vi "Check_Beam_Powers.vi"(3 "Mode":T6, 5 "Traverse line In":T3 {"Row Duration (mins)" format="%#.1f"; "Row No" min=0; "Trace Gas Concentration (%)" min=0.0 format="%#.2f"; "Emission Rate (l/min)" format="%#.2f"; "Tunnel Speed" format="%#.2f"; "Start X" format="%#.2f"; "Start Y" format="%#.2f"; "Start Z" format="%#.2f"; "End X" format="%#.2f"; "End Y" format="%#.2f"; "End Z" format="%#.2f"; "Averaging time (min)" min=0.0 format="%#.2f"}) -> (0 "Error Message":string, 1 "Status":T2, 2 "Traverse line Out":T3 {"Row Duration (mins)" format="%#.1f"; "Row No" min=0; "Trace Gas Concentration (%)" min=0.0 format="%#.2f"; "Emission Rate (l/min)" format="%#.2f"; "Tunnel Speed" format="%#.2f"; "Start X" format="%#.2f"; "Start Y" format="%#.2f"; "Start Z" format="%#.2f"; "End X" format="%#.2f"; "End Y" format="%#.2f"; "End Z" format="%#.2f"; "Averaging time (min)" min=0.0 format="%#.2f"})   [LabVIEW 2012]
uses:
  Gen Trav/Traverse_cluster.ctl
  Gen Trav/Spacing.ctl
  Controls/Multi_run_mode.ctl
  Controls/User_Specific_mode.ctl
  Gen Trav/Multi_Run_Status.ctl
  Controls/Beam_Type.ctl
  Gen Trav/Route mapping/Axis.ctl
  Controls/Setup.ctl
  Controls/Save_Data.ctl
  Globals/Meas_global.vi
  Globals/Extra_Commands_Global.vi
  Globals/LDA_meas_global_1.vi
  Globals/LDA_meas_global_2.vi
panel:
  out "Light Power":dbl=8.10606551e-08 format="%^#_9e"
  in  "stop":bool
  out "Powers":dbl[](array[numeric]) format="%.4f"
  out "Beam Data":dbl[][](array[numeric]) format="%.4f"
  out "Beam Type":T1 items=["Green Unshifted", "Green Shifted", "Blue Unshifted", "Blue Shifted"]
  # "X                      Y                   Z          Datum Power"
  # "Green Unshifted\nGreen Shifted\nBlue Unshifted\nBlue Shifted"
  # "X           Y            Z"
  # "Start"
  # "End"
  # "X           Y            Z"
  # "Start"
  # "End"
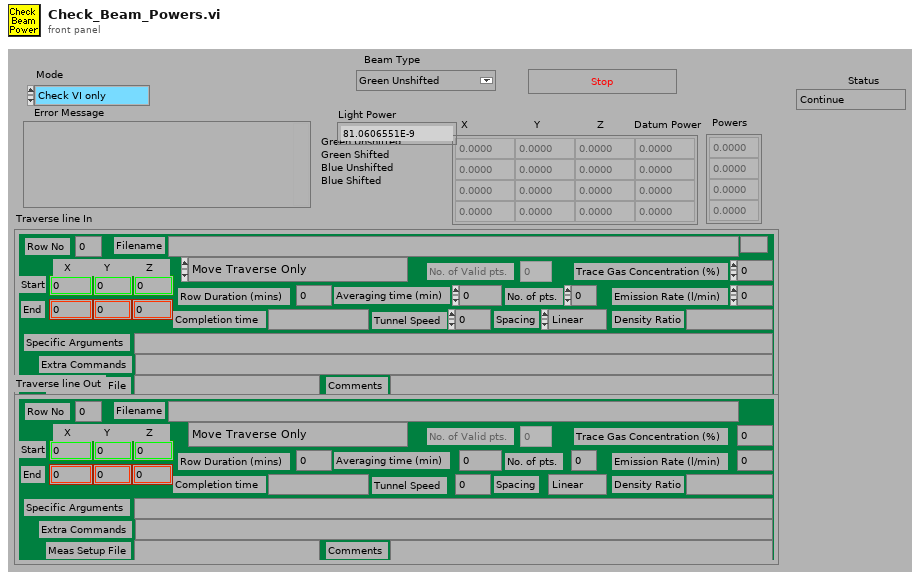
[diagram p1: front panel]
types:
  T1 = typedef "Beam_Type.ctl" = u16
  T2 = typedef "Multi_Run_Status.ctl" = enum16{"Continue", "Jump to Next Point", "Jump to Next Row", "Jump To Fall Back", "Terminate Run"}
  T3 = typedef "Traverse_cluster.ctl" = cluster{"Start X":dbl, "Start Y":dbl, "Start Z":dbl, "End X":dbl, "End Y":dbl, "End Z":dbl, "No. of pts.":i32, "Spacing":T4, "Filename":path, "Tunnel Speed":dbl, "Averaging time (min)":dbl, "Extra Commands":string, "Specific Arguments":string, "Emission Rate (l/min)":dbl, "Trace Gas Concentration (%)":dbl, "Density Ratio":string, "Comments":string, "Row No":i32, "Row Type Selector":T5, "Completion time":string, "Row Duration (mins)":dbl, "No. of Valid pts.":i32, "Meas Setup File":string}
  T4 = typedef "Spacing.ctl" = enum16{"Linear", "Log", "Gauss", "Specified", "N/A"}
  T5 = typedef "Multi_run_mode.ctl" = enum16{"Move Traverse Only", "Set Tunnel Speed Only", "Set Source Only", "Set Measurement Conditions", "Single Measurement", "Vertical Profile", "Lateral Profile", "Longitudinal Profile", "Explore Volume", "Multi-Axis Profile", "Auto Calibrate", "Meas Fast FID Bkgnd", "Check Beam Power", "Scanning Valve Measurement", "Run VI Named:", "Set ADAM Ch", "Wait (minutes)", "Send Message", "Synchronize With:", "Fall Back to this Row", "Turn Off Row Repeating", "Blank Row", "Traverse 3D Volume"}
  T6 = typedef "User_Specific_mode.ctl" = enum16{"Check VI only", "Run VI"}
  T7 = enum32{"Bad", "Idle", "Run top level", "Running"}
  T8 = typedef "LDA_Setup.ctl" = cluster{"dimensions":enum16{"1D", "2D"}, "Analogue Freq Multiplier":dbl}
  T9 = enum16{"Load From Excel File", "Save to Excel File"}
  T10 = typedef "Axis.ctl" = enum16{"X Axis", "X Axis -ve", "Y Axis", "Y Axis -ve", "Z Axis", "Z Axis -ve"}
  T11 = typedef "Save_Data.ctl" = enum16{"Save No Data", "Save Data"}
  T12 = typedef "Setup.ctl" = enum16{"Run Program", "Show Setup", "Save Current Setup", "Setup Front Panel"}
  T13 = typedef "Status_Cluster.ctl" = cluster{"Status":T2, "Error Type":string, "Error Description":string}
  T14 = typedef "BSA_Type.ctl" = enum16{"57N11", "BSA F60"}
  T15 = typedef "BSA_info_Cluster.ctl" = cluster{"GPIB Address":string, "No of Check Bytes":i32, "Extra Info":string, "COLOUR":u32, "Wavelength (nm)":dbl}
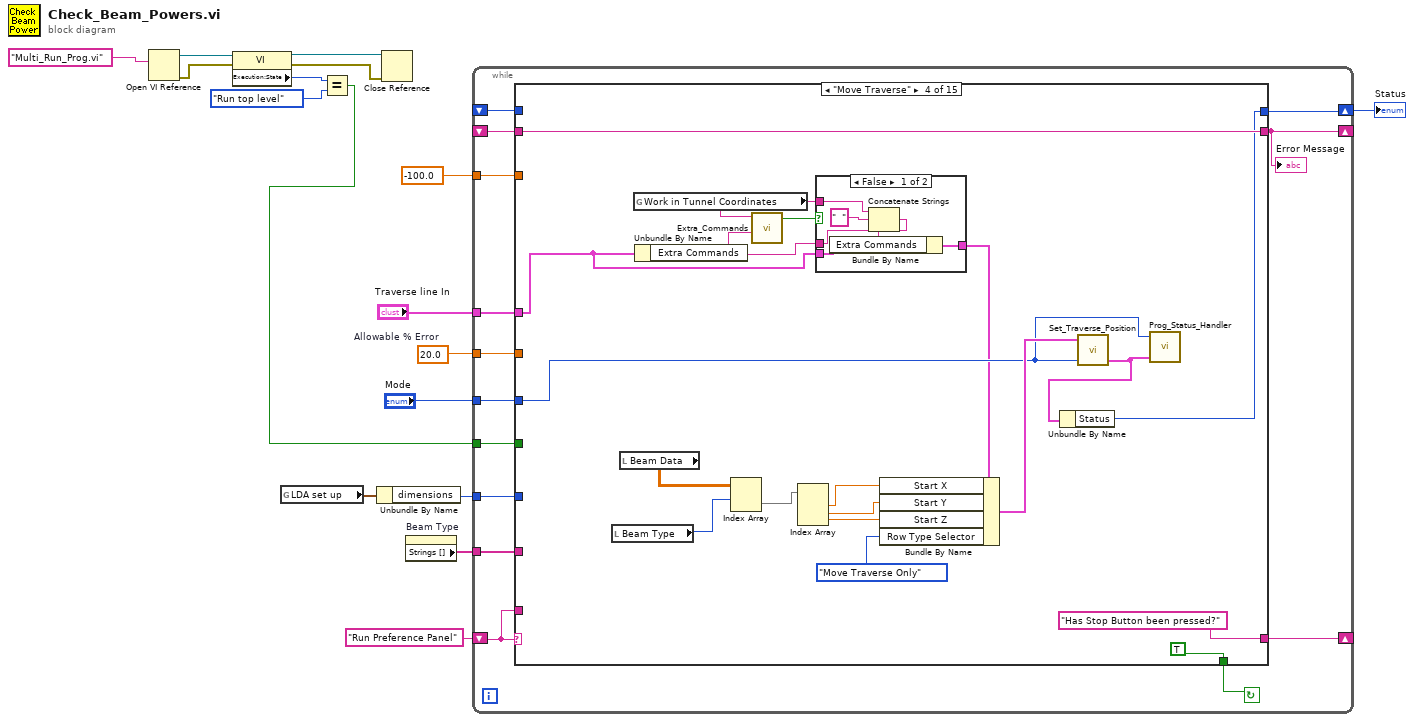
[diagram p0: block diagram]
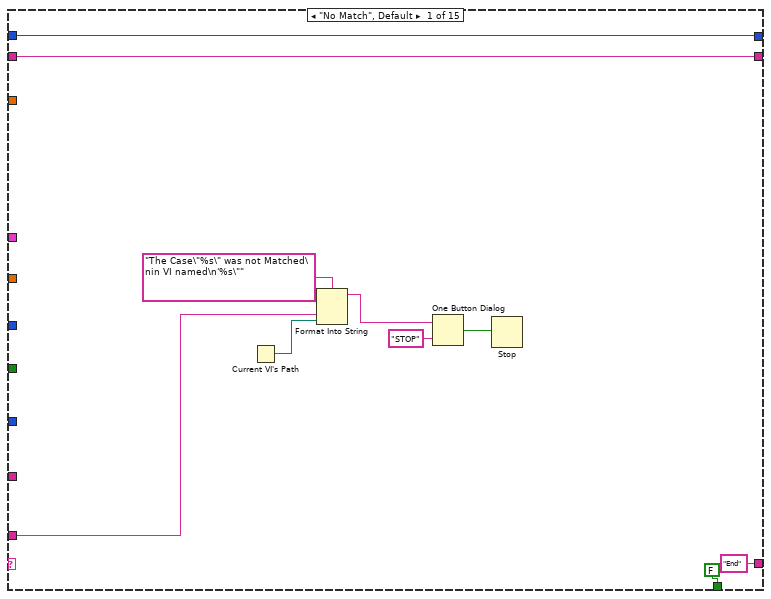
[diagram p2: hidden frame]
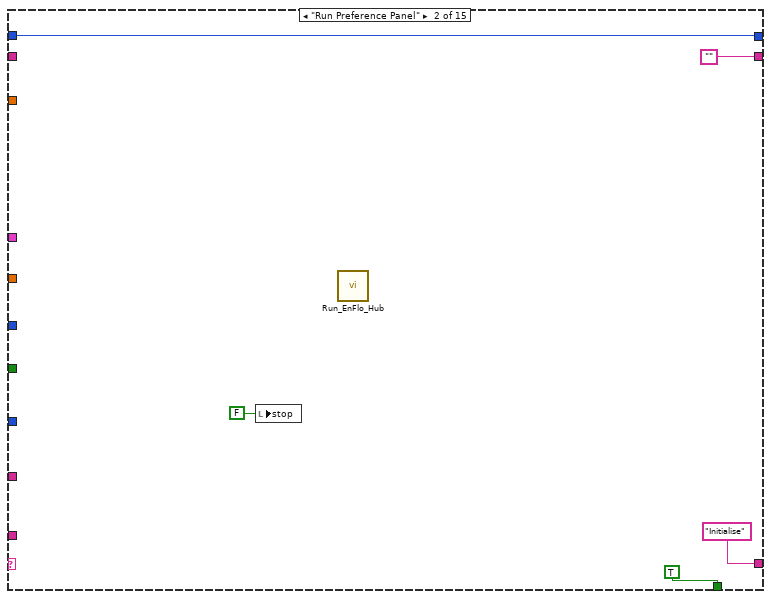
[diagram p3: hidden frame]
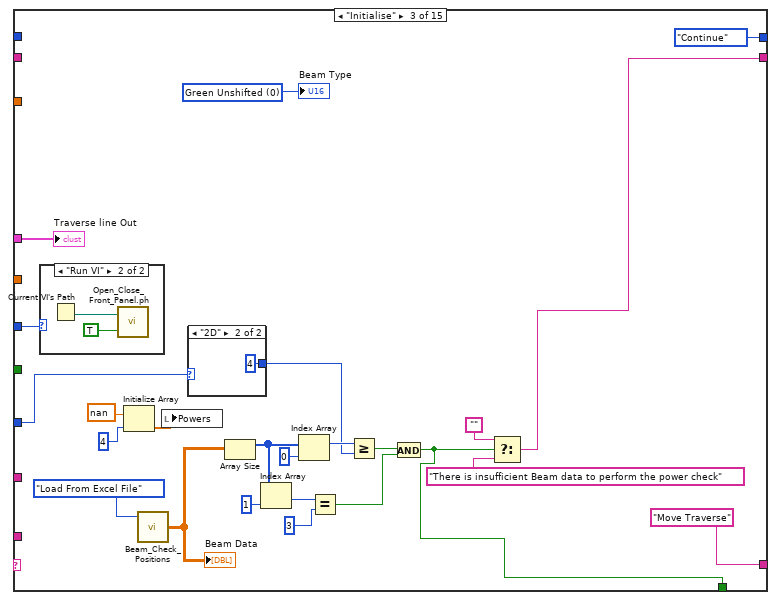
[diagram p4: hidden frame]
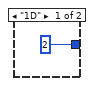
[diagram p5: hidden frame]
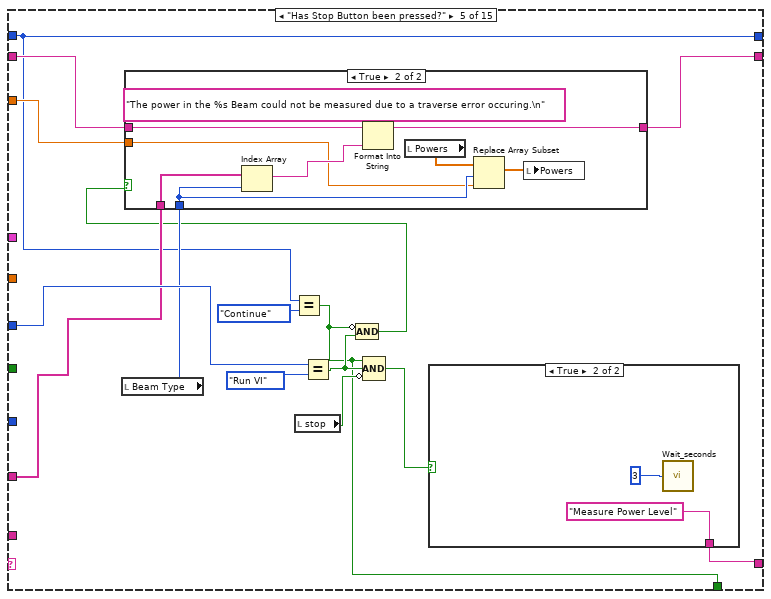
[diagram p8: hidden frame]
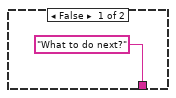
[diagram p10: hidden frame]
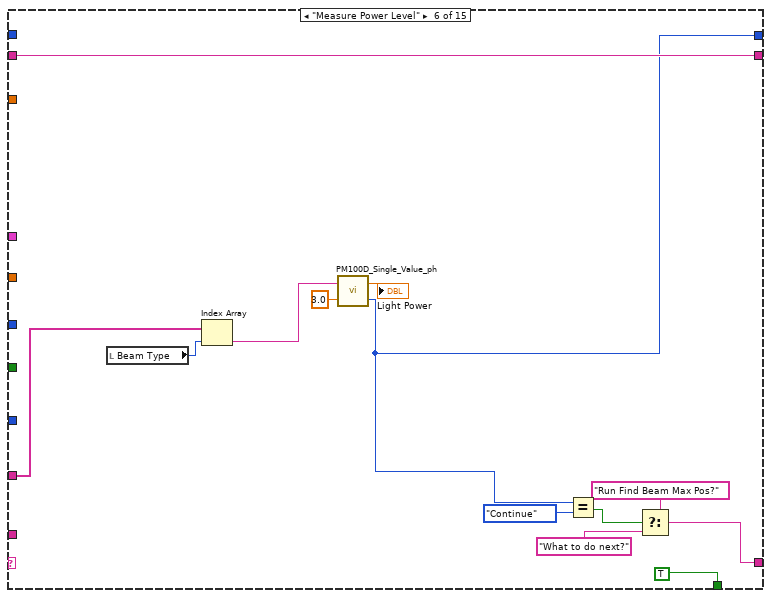
[diagram p11: hidden frame]
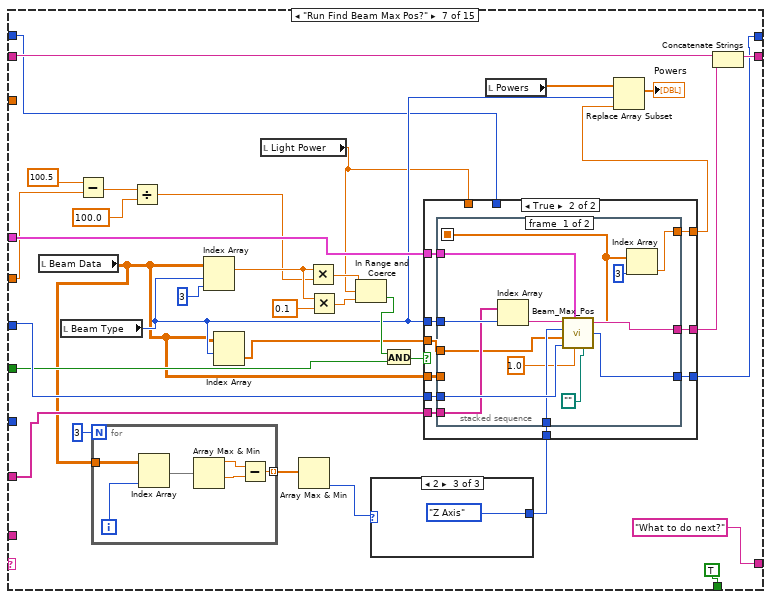
[diagram p12: hidden frame]
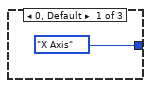
[diagram p13: hidden frame]
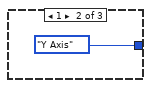
[diagram p14: hidden frame]
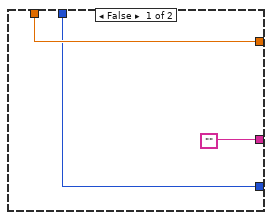
[diagram p15: hidden frame]
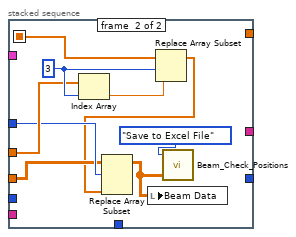
[diagram p16: hidden frame]
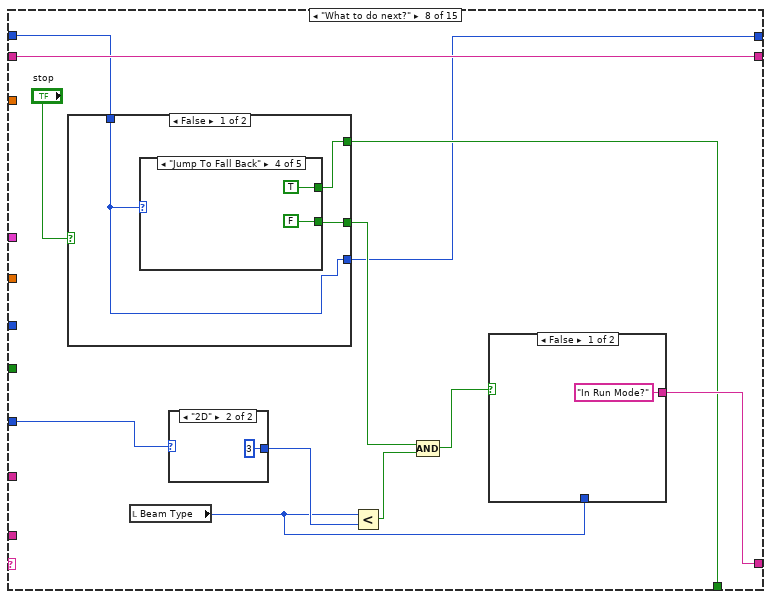
[diagram p17: hidden frame]
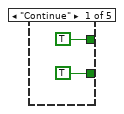
[diagram p18: hidden frame]
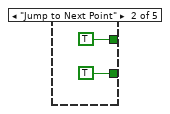
[diagram p19: hidden frame]
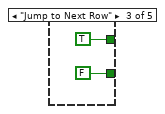
[diagram p20: hidden frame]
diagram:
  w14 = 20.0  # Allowable % Error
  n1 = Open VI Reference(vi path="Multi_Run_Prog.vi") -> (vi reference=w8:refnum<vi>, error out=w9:errorcluster)  [unwired: 1 in, 4 out]
  n2 = property class="VI"(reference=w8, error in=w9) -> (reference out=w10:refnum<vi>, error out=w11:errorcluster, "Execution:State"=w7:T7)
  n3 = global read "Meas_global.vi" "LDA set up"() -> (w2:T8)
  n4 = Equal?(x=w7, y=T7."Run top level" ("Exec.State")) -> (x = y?=w5:bool)
  n5 = Unbundle By Name(w2) -> ("dimensions"=w1:enum16{"1D", "2D"})
  n6 = Close Reference(reference=w10, error in (no error)=w11) -> ()  [unwired: 1 out]
  n7 = property on="Beam Type" class="Ring (strict)"() -> ("Strings []"=w15:string[])  [unwired: 2 in, 2 out]
  n8 = while {
    tunnel: -100.0 ("Element Data") -> [w21]
    tunnel: w14 -> [w23]
    shift-left: _ -> [w25]
    shift-right: [w24] -> _
    tunnel: w1 -> [w26]
    tunnel: w15 -> [w29]
    tunnel: "Traverse line In" -> [w30]
    tunnel: "Mode" -> [w31]
    shift-left: "Run Preference Panel" -> [w22]
    shift-right: [w27] -> _
    tunnel: w5 -> [w20]
    shift-right: [w19] -> w3
    shift-left: _ -> [w18]
    stop <- w28 continue-if-true
    n9 = case shown="\"Move Traverse\"" w22 {
      tunnel: w30 -> [_ _ w68 w76 _ _ w174 _ _ _ _ _ _ w364 _]
      tunnel: w31 -> [_ _ w65 w89 w113 _ w173 _ w262 _ _ _ _ w368 w373]
      tunnel: w29 -> [_ _ _ _ w111 w131 w148 _ _ w279 _ _ _ _ _]
      tunnel: [FALSE ("Update Datum Powers?") TRUE ("Update Datum Powers?") w47 TRUE w102 TRUE TRUE w223 TRUE ("Update Datum Powers?") TRUE TRUE TRUE ("Update Datum Powers?") w334 w365 FALSE ("Update Datum Powers?")] -> w28
      tunnel: ["End" "Initialise" "Move Traverse" "Has Stop Button been pressed?" w112 w136 "What to do next?" w225 w257 "Log Beam Power Readings" w311 "Take datum velocity measurement?" "Move traverse to datum location" "Take a datum velocity measurement" "End"] -> w27
      tunnel: w26 -> [_ _ w64 _ _ _ _ w231 _ _ _ _ w336 _ _]
      tunnel: w25 -> [w33 _ _ w87 w109 w138 w160 w227 w261 w277 w306 w325 w338 w370 w376]
      tunnel: [w33 "" w48 w87 w110 w138 w159 w227 w261 w276 w306 "" w338 w370 w376] -> w24
      tunnel: w23 -> [_ _ _ _ _ _ w156 _ _ _ _ _ _ _ _]
      tunnel: w22 -> [w36 _ _ _ _ _ _ _ _ _ _ _ _ _ _]
      tunnel: w21 -> [_ _ _ _ w108 _ _ _ _ w274 _ _ _ _ _]
      tunnel: w20 -> [_ _ _ _ _ _ w149 _ _ _ _ _ w333 _ _]
      tunnel: [w32 w42 Multi_Run_Status."Continue" ("Status") w84 w101 w133 w143 w221 w255 w273 w309 w321 w331 w363 w372] -> w19
      tunnel: w18 -> [w32 w42 _ _ w101 _ w142 w222 w255 w273 w309 w321 w331 _ w371]
      frame "No Match", Default {
        n10 = Current VI's Path() -> (path=w37:path)
        n11 = Format Into String(format string="The Case\"%s\" was not Matched\nin VI named\n'%s\"" ("Format String"), w36, w37) -> (resulting string=w40:string)  [unwired: 2 in, 1 out]
        n12 = One Button Dialog(message=w40, button name ("OK")="STOP") -> (true=w38:bool)
        n13 = Stop(stop? (T)=w38) -> ()
      }
      frame "Run Preference Panel" {
        n14 = local write "stop"(FALSE ("stop")) -> ()
        n15 = call "Run_EnFlo_Hub.vi"() -> ()  [unwired: 8 out]
      }
      frame "Initialise" {
        w69 = T1 0 items=["Green Unshifted", "Green Shifted", "Blue Unshifted", "Blue Shifted"] ("Beam Type")
        n16 = case shown="\"Run VI\"" w65 {
          frame "Check VI only" {
          }
          frame "Run VI" {
            n17 = Current VI's Path() -> (path=w73:path)
            n18 = call "Open_Close_Front_Panel.ph.vi"("Front Panel Window:Open"=TRUE, "VI path"=w73) -> ()  [unwired: 2 out]
          }
        }
        n19 = Initialize Array(nan ("Numeric"), 4 ("Dimension Size")) -> (w51:dbl[])
        n20 = call "Beam_Check_Positions.vi"("Mode"=T9."Load From Excel File") -> ("Values Out"=w67:dbl[][])  [unwired: 1 in, 1 out]
        "Beam Data" <- w67
        n21 = local write "Powers"(w51) -> ()
        n22 = case shown="\"2D\"" w64 {
          tunnel: [2 4] -> w62
          frame "1D" {
          }
          frame "2D" {
          }
        }
        n23 = Array Size(array=w67) -> (size(s)=w58:i32[])
        n24 = Index Array(array=w58, index=1 ("Index")) -> (element=w57:i32)
        n25 = Index Array(array=w58, index=0 ("Index")) -> (element=w63:i32)
        n26 = Equal?(x=w57, y=3) -> (x = y?=w54:bool)
        n27 = Greater Or Equal?(x=w63, y=w62) -> (x >= y?=w55:bool)
        n28 = And(x=w55, y=w54) -> (x .and. y?=w47:bool)
        n29 = Select(t="", s=w47, f="There is insufficient Beam data to perform the power check") -> (s? t:f=w48:string)
        "Beam Type" <- w69
        "Traverse line Out" <- w68
      }
      frame "Move Traverse" {
        n30 = local read "Beam Type"() -> (w85:T1)
        n31 = local read "Beam Data"() -> (w86:dbl[][])
        n32 = global read "Extra_Commands_Global.vi" "Work in Tunnel Coordinates"() -> (w78:string)
        n33 = Unbundle By Name(w76) -> ("Extra Commands"=w77:string)
        n34 = Index Array(array=w86, index (row)=w85) -> (element=w83:dbl[])  [unwired: 1 in]
        n35 = call "Extra_Commands.vi"("String to Search"=w77, "Command"=w78) -> ("Command Found"=w79:bool)  [unwired: 1 in, 4 out]
        n36 = Index Array(array=w83) -> (element #1=w82:dbl, element #2=w81:dbl, element #3=w80:dbl)  [unwired: 3 in]
        n37 = case shown="False" w79 {
          tunnel: [w99 w100] -> w75
          tunnel: w78 -> [w98 _]
          tunnel: w77 -> [w97 _]
          tunnel: w76 -> [w95 w100]
          frame False {
            n38 = Concatenate Strings(w98, "  " ("string"), w97) -> (w96:string)
            n39 = Bundle By Name(cluster=w95, "Extra Commands"=w96) -> (w99:T3)
          }
          frame True {
          }
        }
        n40 = Bundle By Name(cluster=w75, "Start X"=w82, "Start Y"=w81, "Start Z"=w80, "Row Type Selector"=Multi_run_mode."Move Traverse Only") -> (w92:T3)
        n41 = call "Set_Traverse_Position.vi"("Simulate/Run"=w89, "Traverse line"=w92) -> ("Status Cluster"=w90:T13)  [unwired: 1 in, 2 out]
        n42 = Unbundle By Name(w90) -> ("Status"=w84:T2)
        n43 = call "Prog_Status_Handler.vi"("Status Cluster"=w90, "Simulate/Run"=w89) -> ()  [unwired: 2 out]
      }
      frame "Has Stop Button been pressed?" {
        n44 = local read "Beam Type"() -> (w107:T1)
        n45 = Equal?(x=w101, y=Multi_Run_Status."Continue" ("Status")) -> (x = y?=w102:bool)
        n46 = local read "stop"() -> (w106:bool)
        n47 = Equal?(x=w113, y=User_Specific_mode."Run VI" ("Mode")) -> (x = y?=w104:bool)
        n48 = Compound Arithmetic op=AND(invert w102, w104) -> (w103:bool)
        n49 = case shown="True" w103 {
          tunnel: w107 -> [_ w118]
          tunnel: w111 -> [_ w125]
          tunnel: w109 -> [w116 w122]
          tunnel: [w116 w121] -> w110
          tunnel: w108 -> [_ w117]
          frame False {
          }
          frame True {
            n50 = Index Array(array=w125, index=w118) -> (element=w124:string)
            n51 = Format Into String(format string="The power in the %s Beam could not be measured due to a traverse error occuring.\n" ("Format String"), initial string=w122, w124) -> (resulting string=w121:string)  [unwired: 1 in, 1 out]
            n52 = local read "Powers"() -> (w120:dbl[])
            n53 = Replace Array Subset(array=w120, new element=w117, index=w118) -> (w119:dbl[])
            n54 = local write "Powers"(w119) -> ()
          }
        }
        n55 = Compound Arithmetic op=AND(w102, w104, invert w106) -> (w105:bool)
        n56 = case shown="True" w105 {
          tunnel: ["What to do next?" "Measure Power Level"] -> w112
          frame False {
          }
          frame True {
            n57 = call "Wait_seconds.vi"("Seconds to wait"=u32 3) -> ()
          }
        }
      }
      frame "Measure Power Level" {
        n58 = local read "Beam Type"() -> (w132:T1)
        n59 = Index Array(array=w131, index=w132) -> (element=w130:string)
        n60 = call "PM100D_Single_Value_ph.vi"("Averaging Period (s)"=3.0, "Beam Name"=w130) -> ("Status"=w133:T2, "Light Power mW"=→"Light Power":dbl)
        n61 = Equal?(x=w133, y=Multi_Run_Status."Continue" ("Status")) -> (x = y?=w139:bool)
        n62 = Select(t="Run Find Beam Max Pos?", s=w139, f="What to do next?") -> (s? t:f=w136:string)
      }
      frame "Run Find Beam Max Pos?" {
        n63 = local read "Beam Data"() -> (w145:dbl[][])
        n64 = local read "Beam Type"() -> (w147:T1)
        n65 = Subtract(x=100.5, y=w156) -> (x-y=w155:dbl)
        n66 = for {
          N: 3 -> [_]
          tunnel: w145 -> [w183]
          tunnel: [w179] -> w171 mode=indexing
          i -> [w184]
          n67 = Index Array(array=w183, index (col)=w184) -> (element=w182:dbl[])  [unwired: 1 in]
          n68 = Array Max & Min(array=w182) -> (max value=w181:dbl, min value=w180:dbl)  [unwired: 2 out]
          n69 = Subtract(x=w181, y=w180) -> (x-y=w179:dbl)
        }
        n70 = Divide(x=w155, y=100.0) -> (x/y=w153:dbl)
        n71 = Index Array(array=w145, index (row)=w147, index (col)=3 ("Index")) -> (element=w167:dbl)
        n72 = Index Array(array=w145, index (row)=w147) -> (element=w146:dbl[])  [unwired: 1 in]
        n73 = local read "Light Power"() -> (w144:dbl)
        n74 = Array Max & Min(array=w171) -> (min index (indices)=w170:i32)  [unwired: 3 out]
        n75 = Multiply(x=w167, y=w153) -> (x*y=w165:dbl)
        n76 = Multiply(x=w167, y=0.1) -> (x*y=w164:dbl)
        n77 = In Range and Coerce(upper limit=w165, x=w144, lower limit=w164) -> (In Range?=w151:bool)  [unwired: 1 out]
        n78 = case shown="2" w170 {
          tunnel: [Axis."X Axis" ("Fixed Axis") Axis."Y Axis" ("Fixed Axis") Axis."Z Axis" ("Fixed Axis")] -> w169
          frame 0, Default {
          }
          frame 1 {
          }
          frame 2 {
          }
        }
        n79 = And(x=w151, y=w149) -> (x .and. y?=w150:bool)
        n80 = case shown="True" w150 {
          tunnel: w147 -> [_ w192]
          tunnel: w174 -> [_ w197]
          tunnel: w173 -> [_ w196]
          tunnel: w169 -> [_ w195]
          tunnel: [w187 w194] -> w161
          tunnel: w144 -> [w187 _]
          tunnel: ["" w193] -> w158
          tunnel: w148 -> [_ w191]
          tunnel: w146 -> [_ w190]
          tunnel: w145 -> [_ w189]
          tunnel: [w185 w188] -> w143
          tunnel: w142 -> [w185 _]
          frame False {
          }
          frame True {
            n81 = stacked-sequence {
              seq-local: [w200 _] -> [_ w218]
              tunnel: w197 -> [w211 _]
              tunnel: w196 -> [w210 _]
              tunnel: w195 -> [w209 _]
              tunnel: [w207 _] -> w194
              tunnel: [w206 _] -> w193
              tunnel: w192 -> [w204 w216]
              tunnel: w191 -> [w203 _]
              tunnel: w190 -> [w201 w217]
              tunnel: w189 -> [_ w215]
              tunnel: [w198 _] -> w188
              frame #0 {
                n82 = Index Array(array=w203, index=w204) -> (element=w202:string)
                n83 = call "Beam_Max_Pos.vi"("Picture Log"=path "", "Search Step (mm)"=1.0, "Mode"=w210, "Starting Position"=w201, "Traverse line In"=w211, "Fixed Axis"=w209, "Beam Name"=w202) -> ("Status"=w198:T2, "Beam maxima"=w200:dbl[], "Message"=w206:string)  [unwired: 1 out]
                n84 = Index Array(array=w200, index=3 ("Index")) -> (element=w207:dbl)
              }
              frame #1 {
                w219 = 3 ("index")
                n85 = Index Array(array=w217, index=w219) -> (element=w220:dbl)
                n86 = Replace Array Subset(array=w218, new element=w220, index=w219) -> (w212:dbl[])
                n87 = Replace Array Subset(array=w215, new element=w212, index (row)=w216) -> (w214:dbl[][])  [unwired: 1 in]
                n88 = local write "Beam Data"(w214) -> ()
                n89 = call "Beam_Check_Positions.vi"("Values"=w214, "Mode"=T9."Save to Excel File") -> ()  [unwired: 2 out]
              }
            }
          }
        }
        n90 = local read "Powers"() -> (w163:dbl[])
        n91 = Replace Array Subset(array=w163, new element=w161, index=w147) -> (→"Powers":dbl[])
        n92 = Concatenate Strings(w160, w158) -> (w159:string)
      }
      frame "What to do next?" {
        n93 = case shown="False" "stop" {
          tunnel: [w235 FALSE] -> w224
          tunnel: [w234 FALSE] -> w223
          tunnel: w222 -> [w233 _]
          tunnel: [w233 Multi_Run_Status."Terminate Run" ("Status")] -> w221
          frame False {
            n94 = case shown="\"Jump To Fall Back\"" w233 {
              tunnel: [TRUE TRUE FALSE FALSE FALSE] -> w235
              tunnel: [TRUE TRUE TRUE TRUE FALSE] -> w234
              frame "Continue" {
              }
              frame "Jump to Next Point" {
              }
              frame "Jump to Next Row" {
              }
              frame "Jump To Fall Back" {
              }
              frame "Terminate Run" {
              }
            }
          }
          frame True {
          }
        }
        n95 = local read "Beam Type"() -> (w228:T1)
        n96 = case shown="\"2D\"" w231 {
          tunnel: [1 3] -> w232
          frame "1D" {
          }
          frame "2D" {
          }
        }
        n97 = Less?(x=w228, y=w232) -> (x < y?=w230:bool)
        n98 = Compound Arithmetic op=AND(w224, w230) -> (w229:bool)
        n99 = case shown="False" w229 {
          tunnel: w228 -> [_ w252]
          tunnel: ["In Run Mode?" "Move Traverse"] -> w225
          frame False {
          }
          frame True {
            n100 = Increment(x=w252) -> (x+1=w251:T1)
            n101 = local write "Beam Type"(w251) -> ()
          }
        }
      }
      frame "In Run Mode?" {
        n102 = Equal?(x=w262, y=User_Specific_mode."Run VI" ("Mode")) -> (x = y?=w259:bool)
        n103 = Select(t="Are Powers Acceptable?", s=w259, f="Move traverse to datum location") -> (s? t:f=w257:string)
      }
      frame "Are Powers Acceptable?" {
        n104 = global read "LDA_meas_global_1.vi" "Min Green Unshifted Power mW"() -> (w265:i32)
        n105 = global read "LDA_meas_global_1.vi" "Min Blue Unshifted Power mW"() -> (w267:i32)
        n106 = global read "LDA_meas_global_1.vi" "Min Green Shifted Power mW"() -> (w266:i32)
        n107 = global read "LDA_meas_global_1.vi" "Min Blue Shifted Power mW"() -> (w268:i32)
        n108 = local read "Powers"() -> (w280:dbl[])
        n109 = Build Array(w265, w266, w267, w268) -> (w269:i32[])
        n110 = To Double Precision Float(number=w269) -> (double precision float=w264:dbl[])
        n111 = for {
          tunnel: w280 -> [w287] mode=indexing
          tunnel: w264 -> [w286] mode=indexing
          shift-right: [w296] -> w271
          shift-left: "" -> [w298]
          tunnel: w279 -> [w297] mode=indexing
          tunnel: w274 -> [w291]
          n112 = Subtract(x=w287, y=w286) -> (x-y=w292:dbl)
          n113 = Divide(x=w292, y=w286) -> (x/y=w294:dbl)
          n114 = Not Equal?(x=w291, y=w287) -> (x != y?=w288:bool)
          n115 = Absolute Value(x=w294) -> (abs(x)=w293:dbl)
          n116 = Multiply(x=w293, y=100.0) -> ()  [unwired: 1 out]
          n117 = Less Than 0?(x=w292) -> (x < 0?=w289:bool)
          n118 = Compound Arithmetic op=AND(w288, w289) -> (w290:bool)
          n119 = case shown="True" w290 {
            tunnel: w298 -> [w299 w304]
            tunnel: w297 -> [_ w305]
            tunnel: [w299 w303] -> w296
            tunnel: w287 -> [_ w301]
            tunnel: w286 -> [_ w300]
            frame False {
            }
            frame True {
              n120 = Format Into String(format string="The %s laser beam power is %.1f mW. It lowest acceptable power has been set to %.1f mW. \\n" ("Format String"), initial string=w304, w305, w301, w300) -> (resulting string=w303:string)  [unwired: 1 in, 1 out]
            }
          }
        }
        n121 = Empty String/Path?(string/path=w271) -> (empty?=w272:bool)
        n122 = case shown="False" w272 {
          tunnel: w271 -> [w283 w285]
          tunnel: [w282 w285] -> w270
          frame False {
            n123 = Concatenate Strings(w283, "Please come and check the system As Soon As Possible!\nThe probe may have collided with something or the optical fibres could be getting damaged due to poor launch efficiency! £18,000 TO REPAIR!!\nThe Multi Run will continue." ("Substring")) -> (w282:string)
          }
          frame True {
          }
        }
        n124 = Concatenate Strings(w277, w270) -> (w276:string)
      }
      frame "Log Beam Power Readings" {
        n125 = local read "Beam Data"() -> (w314:dbl[][])
        n126 = local read "Powers"() -> (w313:dbl[])
        n127 = for {
          tunnel: w314 -> [w320] mode=indexing
          tunnel: w313 -> [w317] mode=indexing
          tunnel: [w316] -> w312 mode=indexing
          n128 = Array Subset(array=w320, length=3 ("Array Length")) -> (w318:dbl[])  [unwired: 1 in]
          n129 = Build Array (concatenate)(w318, w317) -> (w316:dbl[])
        }
        n130 = Empty String/Path?(string/path=w306) -> (empty?=w307:bool)
        n131 = call "Log_beam_power.vi"("Message"=w306, "Beam Data"=w312) -> ()  [unwired: 4 out]
        n132 = Select(t="Take datum velocity measurement?", s=w307, f="Send Error Email") -> (s? t:f=w311:string)
      }
      frame "Send Error Email" {
        w329 = FALSE  # Dialog Box (T)
        n133 = Bundle By Name(cluster=errorcluster {"status"=FALSE, "code"=0, "source"=""} ("error in (no error)"), "source"=w325, "status"=TRUE ("Bundle Element")) -> (w327:errorcluster)
        n134 = call "EnFlo_Error_Handler.vi"("error in (no error)"=w327, "Error Type"="Beam Power", "Dialog Box (T)"=w329) -> ()  [unwired: 3 out]
      }
      frame "Take datum velocity measurement?" {
        n135 = global read "LDA_meas_global_1.vi" "BSA Type"() -> (w332:T14)
        n136 = case shown="\"57N11\"" w332 {
          tunnel: w336 -> [w341 _]
          tunnel: [w340 TRUE] -> w335
          tunnel: w333 -> [w339 _]
          frame "57N11" {
            n137 = stacked-sequence {
              tunnel: w341 -> [_ w354]
              tunnel: [_ w350] -> w340
              tunnel: w339 -> [w342 _]
              frame #0 {
                n138 = case shown="True" w342 {
                  frame False {
                  }
                  frame True {
                    n139 = stacked-sequence {
                      frame #0 {
                        n140 = global read "LDA_meas_global_2.vi" "BSA2 info"() -> (w343:T15)
                        n141 = global read "LDA_meas_global_1.vi" "BSA1 info"() -> (w348:T15)
                        n142 = Unbundle By Name(w343) -> ("GPIB Address"=w344:string)
                        n143 = Unbundle By Name(w348) -> ("GPIB Address"=w347:string)
                        n144 = call "Set_BSA_voltage_On_Off.vi"("GPIB address"=w344, "High Voltage"=TRUE) -> ()  [unwired: 1 in, 5 out]
                        n145 = call "Set_BSA_voltage_On_Off.vi"("GPIB address"=w347, "High Voltage"=TRUE) -> ()  [unwired: 1 in, 5 out]
                      }
                      frame #1 {
                        n146 = call "Wait_seconds.vi"("Seconds to wait"=u32 5) -> ()
                      }
                    }
                  }
                }
              }
              frame #1 {
                w351 = 7.0 ("y")
                n147 = call "LDA_data_rate.vi"() -> ("Data rate (Hz) BSA1"=w355:dbl, "Data rate (Hz) BSA2"=w352:dbl)  [unwired: 1 out]
                n148 = Greater?(x=w355, y=w351) -> (0:w353:bool)
                n149 = case shown="\"1D\"" w354 {
                  tunnel: w353 -> [w356 w360]
                  tunnel: w352 -> [_ w359]
                  tunnel: w351 -> [_ w358]
                  tunnel: [w356 w357] -> w350
                  frame "1D" {
                  }
                  frame "2D" {
                    n150 = Greater?(x=w359, y=w358) -> (0:w361:bool)
                    n151 = And(x=w360, y=w361) -> (x .and. y?=w357:bool)
                  }
                }
              }
            }
          }
          frame "BSA F60" {
          }
        }
        n152 = And(x=w335, y=w333) -> (x .and. y?=w334:bool)
      }
      frame "Move traverse to datum location" {
        n153 = call "Set_Traverse_Position.vi"("Simulate/Run"=w368, "Traverse line"=w364) -> ("Status Cluster"=w367:T13)  [unwired: 1 in, 2 out]
        n154 = Unbundle By Name(w367) -> ("Status"=w363:T2)
        n155 = Equal?(x=Multi_Run_Status."Continue" ("Status"), y=w363) -> (x = y?=w365:bool)
      }
      frame "Take a datum velocity measurement" {
        n156 = case shown="\"Run VI\"" w373 {
          tunnel: [w377 w378] -> w372
          tunnel: w371 -> [w377 _]
          frame "Check VI only" {
          }
          frame "Run VI" {
            n157 = flat-sequence {
              tunnel: [w383] -> w380
              tunnel: [w382] -> w379
              tunnel: [w381] -> w378
              tunnel: w380 -> [w391]
              tunnel: w379 -> [w390]
              frame #0 {
                w385 = 1.0  # Averaging time (min)
                w388 = FALSE  # Open Front Panel
                w389 = FALSE  # Remote control
                n158 = call "Create_Error_log_folders.vi"("Log Filename"="LDA_Datum_Vel.xls" ("Input Element")) -> ("Server copy Location"=w382:path, "Local Log File"=w383:path)  [unwired: 2 in, 1 out]
                n159 = call "Code_to_run.vi"("Open Front Panel"=w388, "setup"=Setup."Run Program", "Remote control"=w389, "File"=Save_Data."Save Data", "Results Filename"=w383, "Averaging time (min)"=w385) -> ("Status"=w381:T2)  [unwired: 5 in, 4 out]
              }
              frame #1 {
                n160 = call "Updated_File_Copy.vi"("Target Path"=w390, "Source Path"=w391) -> ()  [unwired: 2 out]
              }
            }
          }
        }
      }
    }
    "Error Message" <- w24
  }
  "Status" <- w3
